vi "DrumSequence_Pulse_Execute.vi"(4 "Set Next Step":bool, 6 "Pass_Through_Time":dbl=-1.0 format="%33.4f", 7 "External Ready":bool=TRUE, 8 "Cancel Time Sec":dbl, 9 "Step Times Sec":dbl[](array[numeric]), 10 "Cancel":bool, 11 "Initiate":bool) -> (0 "Error":bool, 1 "Ready":bool, 2 "Seq  Active":bool, 3 "Step Number State":T1=enum."Initialize")   [LabVIEW 2019, in "Trajectory_Library.lvlib"]
doc: "Implements a simplified state machine similar to a mechanical / electrical drum sequencer. When the Drum Sequencer is \"Ready\" and the \"Initiate\" input becomes TRUE,, the drum sequences through its set of steps from 1 to N. After each Step is executed it is followed by a wait. During the wait the Step output indicates \"Do Nothing\". The number of Steps is determined by the number of elements in the \"Step Times\" input array. Once all the steps have been executed, the Drum Sequencer cycles bac to wait for another initiate. \n\nThere is a Cancel input that interrupts the sequence, executes the Cancel Step, performs the cancel wait, and then returns to wait for an Initiate action. \n\nIf any of the Step Times, or Cancel times are negative, or there more than 32 steps, or less than 1 step an error is signaled. The drum sequencer selects the error state and stays there.\n\nInputs:\n\nOutputs:"
uses:
  Trajectory_Library.lvlib
  Enum/DrumSequence_Step_Enum.ctl
  Enum/DrumSequence_State_Enum.ctl
  Util_GetTime_U32.vi
  Util_GetTime_U64.vi
  <vilib>/Utility/semaphor.llb/Obtain Semaphore Reference.vi
  Timer_Reset.vi
panel:
  # "Time to wait\nafter executing\nstep"
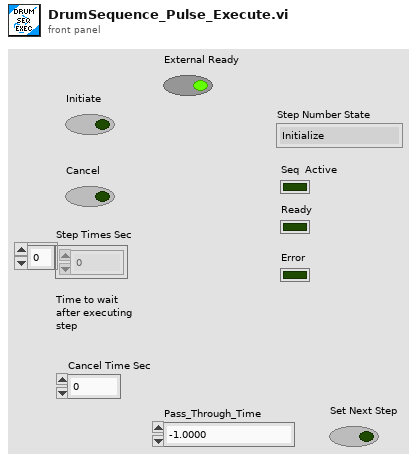
[diagram p1: front panel]
types:
  T1 = typedef "Trajectory_Library.lvlib/DrumSequence_Step_Enum.ctl" = enum16{"Do Nothing", "Step 1", "Step 2", "Step 3", "Step 4", "Step 5", "Step 6", "Step 7", "Step 8", "Step 9", "Step 10", "Step 11", "Step 12", "Step 13", "Step 14", "Step 15", "Step 16", "Step 17", "Step 18", "Step 19", "Step 20", "Step 21", "Step 22", "Step 23", "Step 24", "Step 25", "Step 26", "Step 27", "Step 28", "Step 29", "Step 30", "Step 31", "Step 32", "Cancel", "Initialize", "Error"}
  T2 = typedef "Trajectory_Library.lvlib/DrumSequence_State_Enum.ctl" = enum16{"Initialize", "Ready", "First Step", "Step Wait", "Next State", "Cancel", "Cancel Wait", "Error", "Error Loop"}
  T3 = typedef "Trajectory_Library.lvlib/TIMER.ctl" = cluster{"StartTime":dbl, "Accumulated TIme":dbl, "Running":bool, "semaphore":T4}
  T4 = typedef "Semaphore RefNum" = refnum<k1>
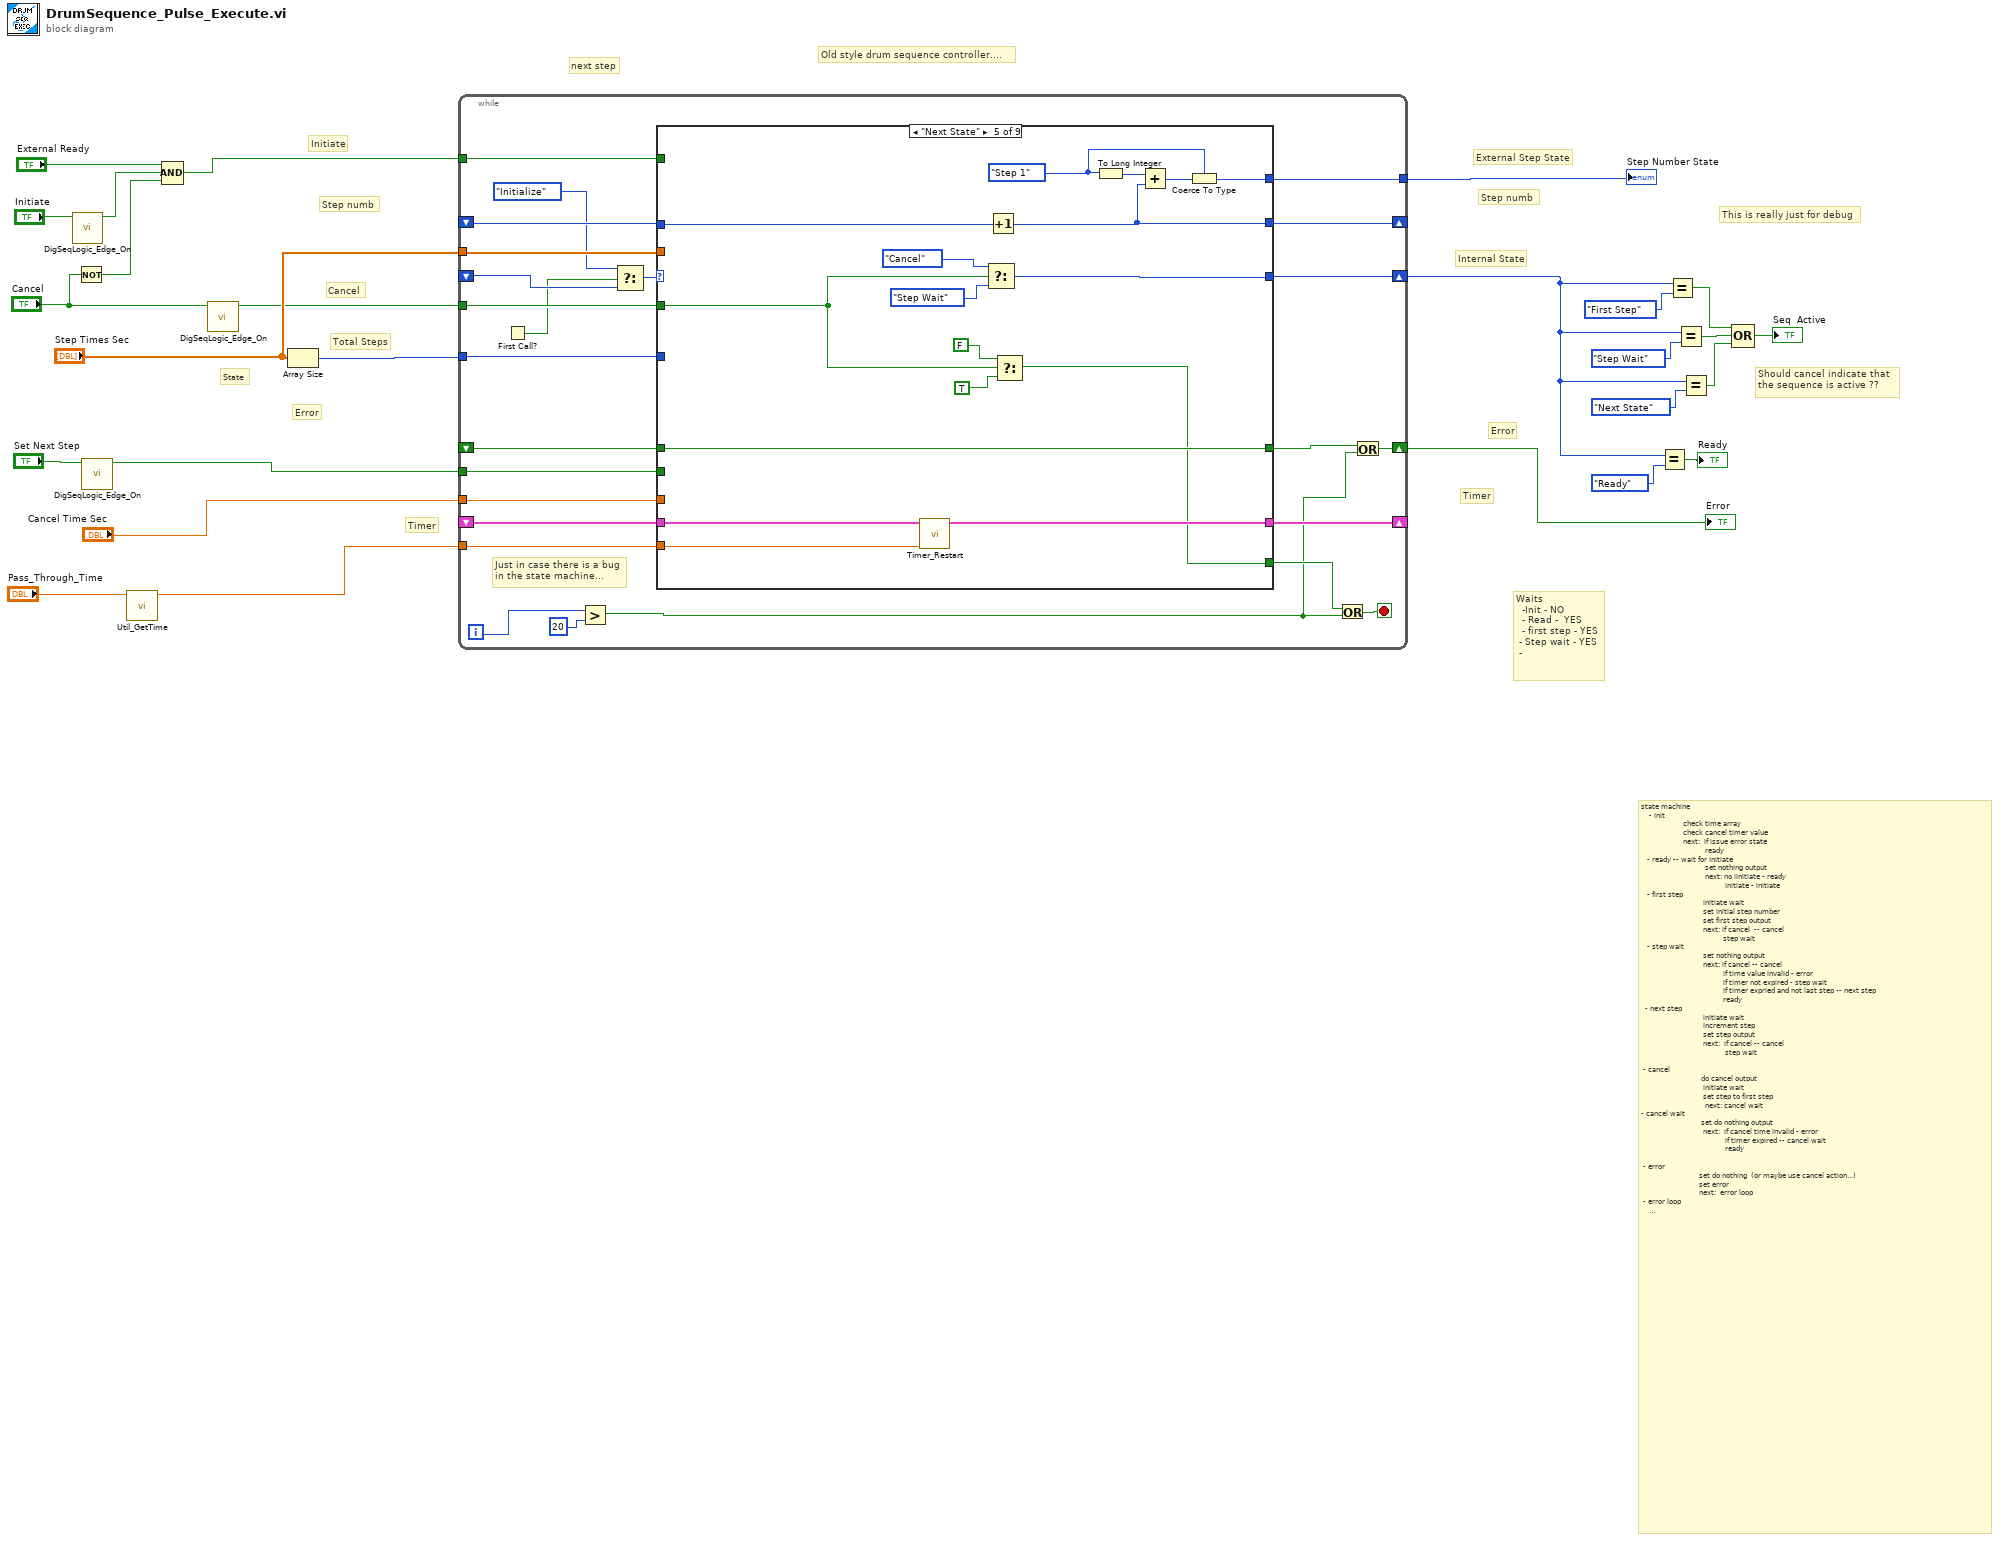
[diagram p0: block diagram]
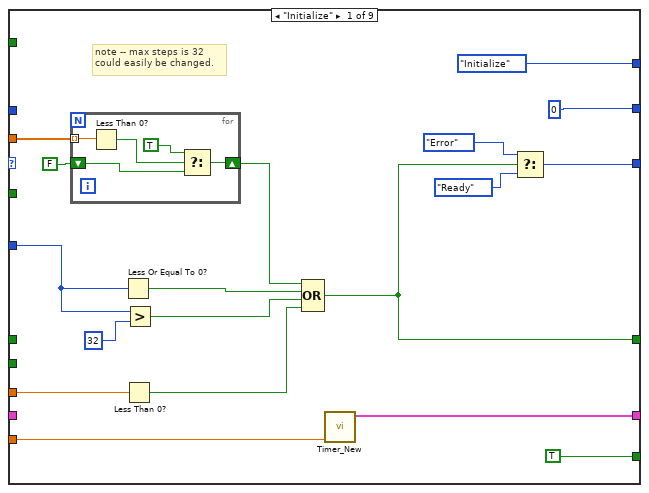
[diagram p2: hidden frame]
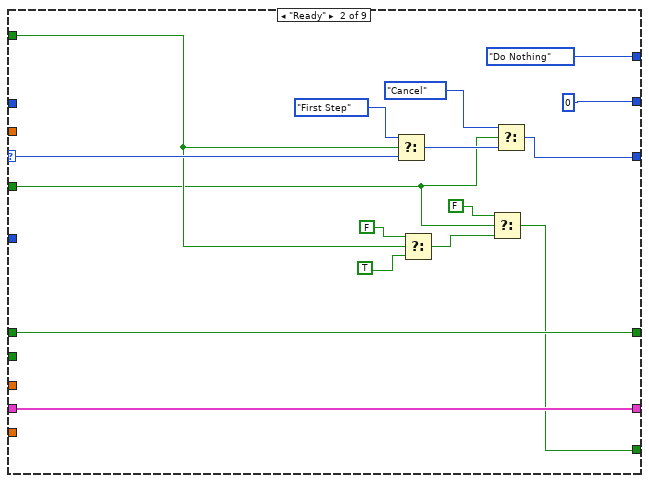
[diagram p3: hidden frame]
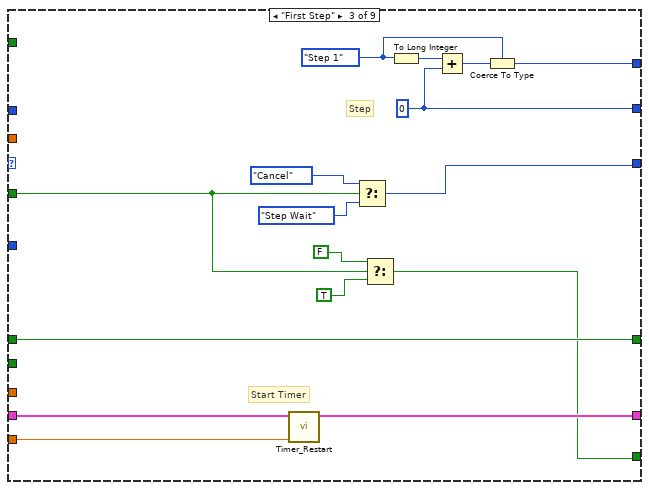
[diagram p4: hidden frame]
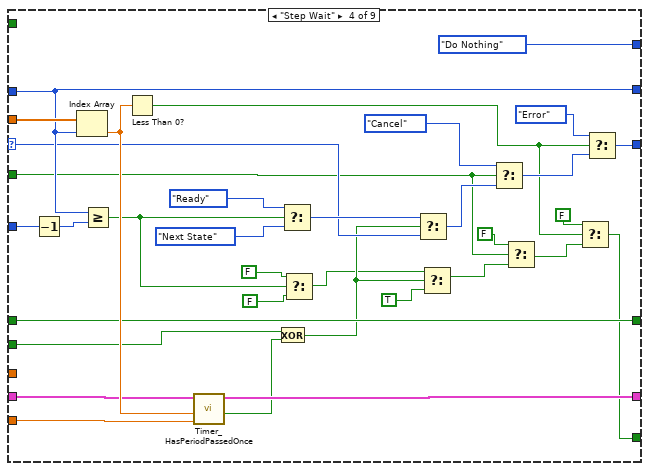
[diagram p5: hidden frame]
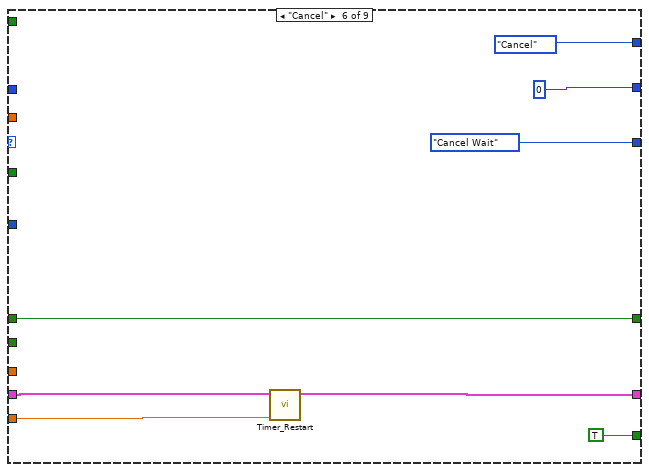
[diagram p6: hidden frame]
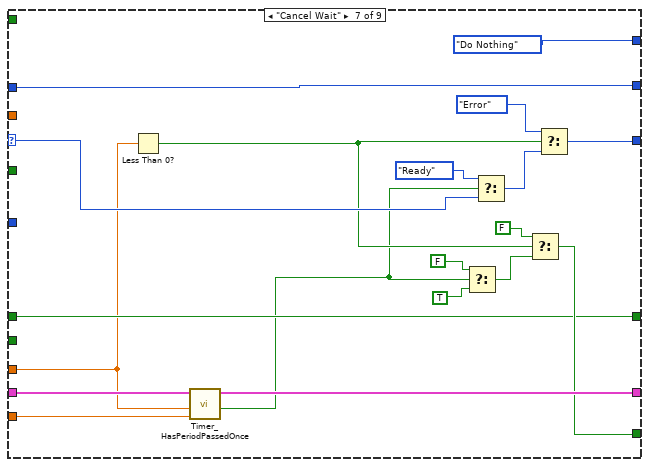
[diagram p7: hidden frame]
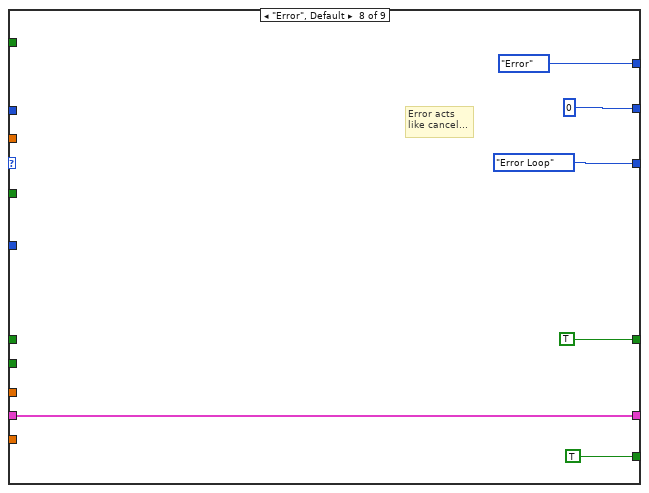
[diagram p8: hidden frame]
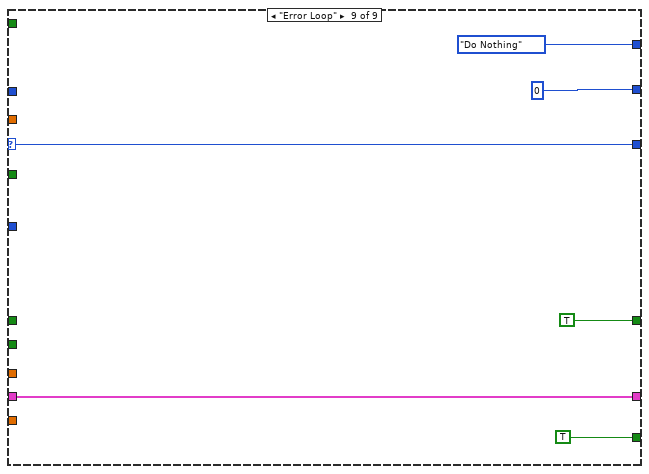
[diagram p9: hidden frame]
diagram:
  # "Should cancel indicate that\nthe sequence is active ??"
  # "This is really just for debug"
  # "Waits\n  -Init - NO\n  - Read -  YES\n  - first step - YES\n - Step wait - YES\n -"
  # "Timer"
  # "Error"
  # "State"
  # "Total Steps"
  # "Cancel"
  # "Step numb"
  # "Initiate"
  # "next step"
  # "Old style drum sequence controller...."
  # "Step numb"
  # "Timer"
  # "Error"
  # "Internal State"
  # "External Step State"
  # "state machine\n    - init\n                     check time array\n                     check cancel timer value\n                     next:  if issue error state\n                                ready\n   - ready -- wait for initiate\n                                set nothing output\n                                next: no iinitiate - ready\n                                          initiate - initiate\n   - first step \n                               initiate wait\n                               set initial step number\n                               set first step output\n                               next: if cancel  -- cancel\n                                         step wait\n   - step wait \n                               set nothing output\n                               next: if cancel -- cancel\n                                         if time value invalid - error\n                                         if timer not expired - step wait\n                                         if timer expried and not last step -- next step\n                                         ready\n  - next step\n                               initiate wait\n                               increment step\n                               set step output\n                               next:  if cancel -- cancel\n                                          step wait\n\n - cancel\n                              do cancel output\n                               initiate wait\n                               set step to first step\n                                next: cancel wait\n- cancel wait\n                              set do nothing output\n                               next:  if cancel time invalid - error\n                                          if timer expired -- cancel wait\n                                          ready\n\n - error\n                             set do nothing  (or maybe use cancel action...)\n                             set error\n                             next:  error loop\n - error loop\n                             set do nothing\n                             set error\n                             next: error loop"
  n1 = call "DigSeqLogic_Edge_On.vi"("Input"="Initiate") -> ("On Edge"=w24:bool)  [unwired: 10 in]
  n2 = Not(x="Cancel") -> (.not. x?=w26:bool)
  n3 = call "DigSeqLogic_Edge_On.vi"("Input"="Set Next Step") -> ("On Edge"=w4:bool)  [unwired: 10 in]
  n4 = call "Util_GetTime.vi"("Pass_Through_Time"="Pass_Through_Time") -> ("FPGA_Time_Seconds"=w19:dbl)  [unwired: 8 in, 2 out]
  n5 = Compound Arithmetic op=AND("External Ready", w24, w26) -> (w18:bool)
  n6 = call "DigSeqLogic_Edge_On.vi"("Input"="Cancel") -> ("On Edge"=w1:bool)  [unwired: 10 in]
  n7 = Array Size(array="Step Times Sec") -> (size(s)=w23:i32)
  n8 = while {
    tunnel: "Step Times Sec" -> [w50]
    tunnel: "Cancel Time Sec" -> [w49]
    tunnel: w19 -> [w48]
    tunnel: w18 -> [w47]
    tunnel: w1 -> [w46]
    tunnel: [w43] -> w7
    tunnel: w4 -> [w42]
    tunnel: w23 -> [w51]
    shift-right: [w41] -> _
    shift-left: _ -> [w35]
    shift-right: [w29] -> w3
    shift-left: _ -> [w40]
    shift-right: [w44] -> w8
    shift-left: _ -> [w37]
    shift-right: [w45] -> _
    shift-left: _ -> [w39]
    i -> [w31]
    stop <- w33 stop-if-true
    # "Just in case there is a bug\nin the state machine..."
    n9 = First Call?() -> (First Call?: T/F=w34:bool)
    n10 = Greater?(x=w31, y=20) -> (0:w27:bool)
    n11 = Select(t=DrumSequence_State_Enum."Initialize", s=w34, f=w37) -> (s? t:f=w38:T2)
    n12 = case shown="\"Next State\"" w38 {
      selector: w38 -> [_ w89 _ w127 _ _ w178 _ w195]
      tunnel: w51 -> [w58 _ _ w125 _ _ _ _ _]
      tunnel: w50 -> [w68 _ _ w133 _ _ _ _ _]
      tunnel: w49 -> [w67 _ _ _ _ _ w167 _ _]
      tunnel: [w64 w86 w96 w120 w143 w160 w170 TRUE TRUE] -> w28
      tunnel: [w61 w79 w91 w130 w150 DrumSequence_State_Enum."Cancel Wait" w181 DrumSequence_State_Enum."Error Loop" w195] -> w44
      tunnel: [w60 w85 w101 w139 w148 w163 w182 w185 w192] -> w41
      tunnel: w48 -> [w59 _ w102 w140 w149 w164 w169 _ _]
      tunnel: [DrumSequence_Step_Enum."Initialize" ("Step Number") DrumSequence_Step_Enum."Do Nothing" ("Step Number") w104 DrumSequence_Step_Enum."Do Nothing" ("Step Number") w151 DrumSequence_Step_Enum."Cancel" ("Step Number") DrumSequence_Step_Enum."Do Nothing" ("Step Number") DrumSequence_Step_Enum."Error" ("Step Number") DrumSequence_Step_Enum."Do Nothing" ("Step Number")] -> w43
      tunnel: w47 -> [_ w84 _ _ _ _ _ _ _]
      tunnel: [0 0 w103 w128 w152 0 w179 0 0] -> w45
      tunnel: w46 -> [_ w76 w95 w112 w144 _ _ _ _]
      tunnel: w39 -> [_ _ _ w128 w153 _ w179 _ _]
      tunnel: w42 -> [_ _ _ w122 _ _ _ _ _]
      tunnel: w35 -> [_ w85 w97 w121 w142 w158 w168 w185 w192]
      tunnel: w40 -> [_ w86 w96 w120 w143 w160 w170 _ _]
      tunnel: [TRUE w75 w92 w107 w141 TRUE w172 TRUE TRUE] -> w32
      frame "Initialize" {
        # "note -- max steps is 32\ncould easily be changed."
        n13 = for {
          shift-right: [w73] -> w66
          shift-left: FALSE -> [w72]
          tunnel: w68 -> [w74] mode=indexing
          n14 = Less Than 0?(x=w74) -> (x < 0?=w70:bool)
          n15 = Select(t=TRUE, s=w70, f=w72) -> (s? t:f=w73:bool)
        }
        n16 = Less Or Equal To 0?(x=w58) -> (x <= 0?=w65:bool)
        n17 = Less Than 0?(x=w67) -> (x < 0?=w52:bool)
        n18 = Greater?(x=w58, y=32) -> (0:w53:bool)
        n19 = Compound Arithmetic op=OR(w66, w65, w53, w52) -> (w64:bool)
        n20 = call "Timer_New.vi"("Pass_Through_Time"=w59) -> ("TIMER"=w60:T3)  [unwired: 10 in]
        n21 = Select(t=DrumSequence_State_Enum."Error", s=w64, f=DrumSequence_State_Enum."Ready") -> (s? t:f=w61:T2)
      }
      frame "Ready" {
        n22 = Select(t=DrumSequence_State_Enum."First Step", s=w84, f=w89) -> (s? t:f=w80:T2)
        n23 = Select(t=FALSE, s=w84, f=TRUE) -> (s? t:f=w77:bool)
        n24 = Select(t=FALSE, s=w76, f=w77) -> (s? t:f=w75:bool)
        n25 = Select(t=DrumSequence_State_Enum."Cancel", s=w76, f=w80) -> (s? t:f=w79:T2)
      }
      frame "First Step" {
        w98 = DrumSequence_Step_Enum."Step 1" ("Step Number")
        w103 = 0
        # "Start Timer"
        # "Step"
        n26 = call "Timer_Restart.vi"("Pass_Through_Time"=w102, "in Timer"=w97) -> ("out Timer"=w101:T3)  [unwired: 9 in]
        n27 = Select(t=DrumSequence_State_Enum."Cancel", s=w95, f=DrumSequence_State_Enum."Step Wait") -> (s? t:f=w91:T2)
        n28 = Select(t=FALSE, s=w95, f=TRUE) -> (s? t:f=w92:bool)
        n29 = To Long Integer(number=w98) -> (32bit integer=w106:i32)
        n30 = Add(x=w106, y=w103) -> (x+y=w105:i32)
        n31 = Coerce To Type(0:w105, 1:w98) -> (2:w104:T1)
      }
      frame "Step Wait" {
        n32 = Decrement(x=w125) -> (x-1=w126:i32)
        n33 = Index Array(array=w133, index=w128) -> (element=w132:dbl)
        n34 = Greater Or Equal?(x=w128, y=w126) -> (x >= y?=w119:bool)
        n35 = Less Than 0?(x=w132) -> (x < 0?=w108:bool)
        n36 = call "Timer_HasPeriodPassedOnce.vi"("Pass_Through_Time"=w140, "Period"=w132, "in Timer"=w121) -> ("Expired"=w123:bool, "out Timer"=w139:T3)  [unwired: 6 in, 1 out]
        n37 = Exclusive Or(1:w123, 2:w122) -> (0:w116:bool)
        n38 = Select(t=DrumSequence_State_Enum."Ready", s=w119, f=DrumSequence_State_Enum."Next State") -> (s? t:f=w134:T2)
        n39 = Select(t=FALSE, s=w119, f=FALSE) -> (s? t:f=w115:bool)
        n40 = Select(t=w134, s=w116, f=w127) -> (s? t:f=w137:T2)
        n41 = Select(t=w115, s=w116, f=TRUE) -> (s? t:f=w113:bool)
        n42 = Select(t=DrumSequence_State_Enum."Cancel", s=w112, f=w137) -> (s? t:f=w129:T2)
        n43 = Select(t=FALSE, s=w112, f=w113) -> (s? t:f=w109:bool)
        n44 = Select(t=FALSE, s=w108, f=w109) -> (s? t:f=w107:bool)
        n45 = Select(t=DrumSequence_State_Enum."Error", s=w108, f=w129) -> (s? t:f=w130:T2)
      }
      frame "Next State" {
        w147 = DrumSequence_Step_Enum."Step 1" ("Step Number")
        n46 = call "Timer_Restart.vi"("Pass_Through_Time"=w149, "in Timer"=w142) -> ("out Timer"=w148:T3)  [unwired: 9 in]
        n47 = Select(t=DrumSequence_State_Enum."Cancel", s=w144, f=DrumSequence_State_Enum."Step Wait") -> (s? t:f=w150:T2)
        n48 = Increment(x=w153) -> (x+1=w152:i32)
        n49 = Select(t=FALSE, s=w144, f=TRUE) -> (s? t:f=w141:bool)
        n50 = To Long Integer(number=w147) -> (32bit integer=w157:i32)
        n51 = Add(x=w157, y=w152) -> (x+y=w156:i32)
        n52 = Coerce To Type(0:w156, 1:w147) -> (2:w151:T1)
      }
      frame "Cancel" {
        n53 = call "Timer_Restart.vi"("Pass_Through_Time"=w164, "in Timer"=w158) -> ("out Timer"=w163:T3)  [unwired: 9 in]
      }
      frame "Cancel Wait" {
        n54 = Less Than 0?(x=w167) -> (x < 0?=w171:bool)
        n55 = call "Timer_HasPeriodPassedOnce.vi"("Pass_Through_Time"=w169, "Period"=w167, "in Timer"=w168) -> ("Expired"=w166:bool, "out Timer"=w182:T3)  [unwired: 6 in, 1 out]
        n56 = Select(t=FALSE, s=w166, f=TRUE) -> (s? t:f=w176:bool)
        n57 = Select(t=DrumSequence_State_Enum."Ready", s=w166, f=w178) -> (s? t:f=w183:T2)
        n58 = Select(t=FALSE, s=w171, f=w176) -> (s? t:f=w172:bool)
        n59 = Select(t=DrumSequence_State_Enum."Error", s=w171, f=w183) -> (s? t:f=w181:T2)
      }
      frame "Error", Default {
        # "Error acts\nlike cancel..."
      }
      frame "Error Loop" {
      }
    }
    n60 = Or(x=w32, y=w27) -> (x .or. y?=w33:bool)
    n61 = Or(x=w28, y=w27) -> (x .or. y?=w29:bool)
  }
  "Error" <- w3
  "Step Number State" <- w7
  n62 = Equal?(x=w8, y=DrumSequence_State_Enum."Ready") -> (x = y?=→"Ready":bool)
  n63 = Equal?(x=w8, y=DrumSequence_State_Enum."First Step") -> (x = y?=w12:bool)
  n64 = Equal?(x=w8, y=DrumSequence_State_Enum."Step Wait") -> (x = y?=w11:bool)
  n65 = Equal?(x=w8, y=DrumSequence_State_Enum."Next State") -> (x = y?=w10:bool)
  n66 = Compound Arithmetic op=OR(w12, w11, w10) -> (→"Seq  Active":bool)
